vi "Should Show PSD Window.vi"(11 "Data in":T1={"First Time"=FALSE, "Show PSD Window"=FALSE, "Show PSD Window Clicked"=FALSE, "Export mode"=0, "Window"=1, "dB"=FALSE, "Averaging parameters"={"averaging mode"=enum."No averaging", "weighting mode"=enum."Exponential", "number of averages"=10}, "Window parameter"=nan, "Number of Samples"=1000, "PSD VI Ref"=refnum} {"Averaging parameters"."number of averages" min=1; "Window" items=["Rectangle"=0, "Hanning"=1, "Hamming"=2, "Blackman-Harris"=3, "Exact Blackman"=4, "Blackman"=5, "Flat Top"=6, "4 Term B-Harris "=7, "7 Term B-Harris"=8, "Low Sidelobe"=9, "Blackman Nuttall"=11, "Triangle"=30, "Bartlett-Hanning"=31, "Bohman"=32, "Parzen"=33, "Welch"=34, "Kaiser"=60, "Dolph-Chebyshev"=61, "Gaussian"=62]; "Export mode" items=["Power Spectrum", "Power Spectral Density"]}) -> (2 "Show window":bool, 3 "Data out":T1={"First Time"=FALSE, "Show PSD Window"=FALSE, "Show PSD Window Clicked"=FALSE, "Export mode"=0, "Window"=1, "dB"=FALSE, "Averaging parameters"={"averaging mode"=enum."No averaging", "weighting mode"=enum."Exponential", "number of averages"=10}, "Window parameter"=nan, "Number of Samples"=1000, "PSD VI Ref"=refnum} {"Averaging parameters"."number of averages" min=1; "Window" items=["Rectangle"=0, "Hanning"=1, "Hamming"=2, "Blackman-Harris"=3, "Exact Blackman"=4, "Blackman"=5, "Flat Top"=6, "4 Term B-Harris "=7, "7 Term B-Harris"=8, "Low Sidelobe"=9, "Blackman Nuttall"=11, "Triangle"=30, "Bartlett-Hanning"=31, "Bohman"=32, "Parzen"=33, "Welch"=34, "Kaiser"=60, "Dolph-Chebyshev"=61, "Gaussian"=62]; "Export mode" items=["Power Spectrum", "Power Spectral Density"]})   [LabVIEW 2023, in "Power Spectrum Density.lvlib" / "Power Spectrum Density.lvclass"]
uses:
  Power Spectrum Density.lvclass
  Power Spectrum Density Data.ctl
  <vilib>/measure/maspectr.llb/Power Spectrum and PSD Export Mode.ctl
  <vilib>/Analysis/4window.llb/windowTd.ctl
  <vilib>/measure/NI_MAPro.lvlib
  <vilib>/Analysis/NI_AALPro.lvlib
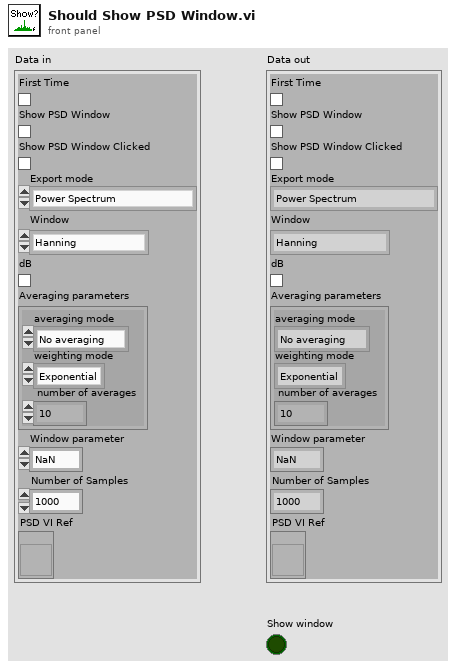
[diagram p1: front panel]
types:
  T1 = typedef "Power Spectrum Density.lvlib/Power Spectrum Density.lvclass/Power Spectrum Density Data.ctl" = cluster{"First Time":bool, "Show PSD Window":bool, "Show PSD Window Clicked":bool, "Export mode":T2, "Window":T3, "dB":bool, "Averaging parameters":cluster{"averaging mode":enum16{"No averaging", "Vector averaging", "RMS averaging", "Peak hold"}, "weighting mode":enum16{"Linear", "Exponential"}, "number of averages":u32}, "Window parameter":dbl, "Number of Samples":i32, "PSD VI Ref":refnum<vi>}
  T2 = typedef "NI_MAPro.lvlib/Power Spectrum and PSD Export Mode.ctl" = u16
  T3 = typedef "NI_AALPro.lvlib/windowTd.ctl" = u32
  T4 = enum32{"Invalid", "Standard", "Closed", "Hidden", "Minimized", "Maximized"}
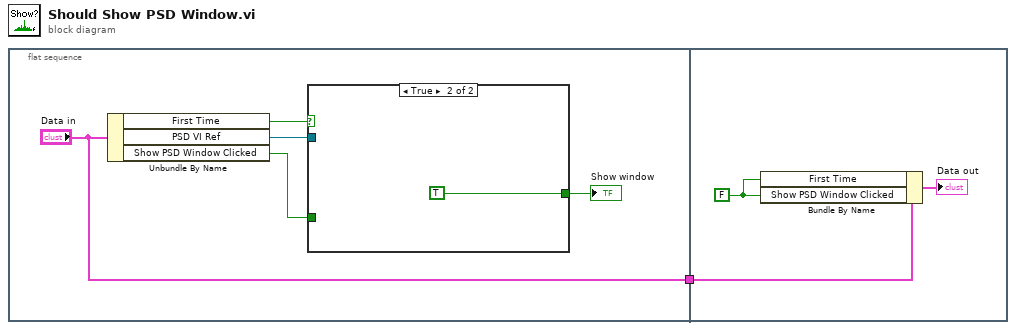
[diagram p0: block diagram]
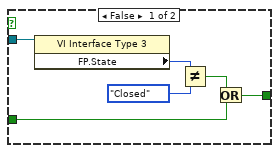
[diagram p2: hidden frame]
diagram:
  n1 = flat-sequence {
    tunnel: ["Data in"] -> w1
    tunnel: w1 -> [w16]
    frame #0 {
      n2 = Unbundle By Name("Data in") -> ("First Time"=w4:bool, "PSD VI Ref"=w6:refnum<vi>, "Show PSD Window Clicked"=w5:bool)
      n3 = case shown="True" w4 {
        tunnel: w6 -> [w12 _]
        tunnel: [w7 TRUE] -> w2
        tunnel: w5 -> [w9 _]
        frame False {
          n4 = property class="VI Interface Type 3"(reference=w12) -> ("FP.State"=w11:T4)  [unwired: 1 in, 2 out]
          n5 = Not Equal?(x=w11, y=T4."Closed" ("Front Panel Window:State")) -> (x != y?=w8:bool)
          n6 = Or(x=w8, y=w9) -> (x .or. y?=w7:bool)
        }
        frame True {
        }
      }
      "Show window" <- w2
    }
    frame #1 {
      w14 = FALSE ("Show Spectrogram Window Button Clicked")
      n7 = Bundle By Name(cluster=w16, "First Time"=w14, "Show PSD Window Clicked"=w14) -> (→"Data out":T1)
    }
  }
